vi "RT Driver VI.vi"(7 "Operation":T1, 11 "Device Reference in":T2 format="%.0x") -> (0 "Error Code":i32)   [LabVIEW 2020, in "FlexRay Custom Device Engine.lvlib"]
uses:
  FlexRay Custom Device Engine.lvlib
  <vilib>/NI VeriStand/Custom Device API/Custom Device Item Ref.ctl
  <vilib>/NI VeriStand/Custom Device API/Hardware Interface Driver VI Operation.ctl
  <vilib>/NI VeriStand/Custom Device API/Data Reference.ctl
  Shared/FREventInfo.ctl
  Shared/InterfaceState.ctl
  <vilib>/xnet/xnet.llb/XNET Control Scope.ctl
  <vilib>/NI VeriStand/Custom Device API/Global Data Refs.vi
  <vilib>/xnet/xnet.llb/XNET Read (State FlexRay Comm).vi
  <vilib>/NI VeriStand/Custom Device API/Custom Device API.lvlib
  Shared/FlexRay Custom Device Shared.lvlib
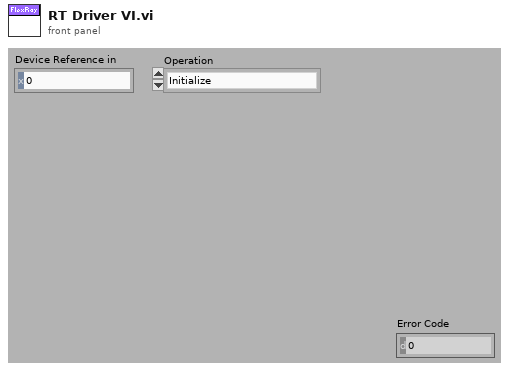
[diagram p1: front panel]
types:
  T1 = typedef "Custom Device API.lvlib/Hardware Interface Driver VI Operation.ctl" = enum16{"Initialize", "Start", "Read Data from HW", "Write Data to HW", "Close"}
  T2 = typedef "Custom Device API.lvlib/Custom Device Item Ref.ctl" = u64
  T3 = typedef "Custom Device API.lvlib/Data Reference.ctl" = i32
  T4 = typedef "FlexRay Custom Device Shared.lvlib/FREventInfo.ctl" = cluster{"Signals":refnum<k21>[], "Channel Data Ref":T3[], "Channel Data Value":dbl[]}
  T5 = typedef "FlexRay Custom Device Engine.lvlib/InterfaceState.ctl" = enum16{"Disabled", "Enabled", "Init"}
  T6 = cluster{"ctrl_stat":cluster{"ctrl_state":T2[], "FR Intf":refnum<k21>}, "FRConfig":cluster{"Write signal list":refnum<k21>[], "Output Values":dbl[], "Output Refs":T3[], "Read signal list":refnum<k21>[], "Input Values":dbl[], "Input Refs":T3[], "EventFrames list":T4[], "FR Cyclic Session":refnum<k21>, "FR Single Read Session":refnum<k21>, "FR Event Write Sessions":refnum<k21>[], "Run state":T5}, "ActiveCom":cluster{"CyclicFRActive?":bool, "EventFRActive?":bool, "IncomingFRActive?":bool}, "Device Error":errorcluster}
  T7 = typedef "XNET Control Scope.ctl" = u32
  T8 = typedef "XNET FlexRay Comm.ctl" = cluster{"fault code":i32, "fault?":bool, "FlexRay POC state":T9, "clock correction failed":u8, "passive to active count":u8, "channel A sleep?":bool, "channel B sleep?":bool}
  T9 = typedef "XNET FlexRay POC State.ctl" = u8
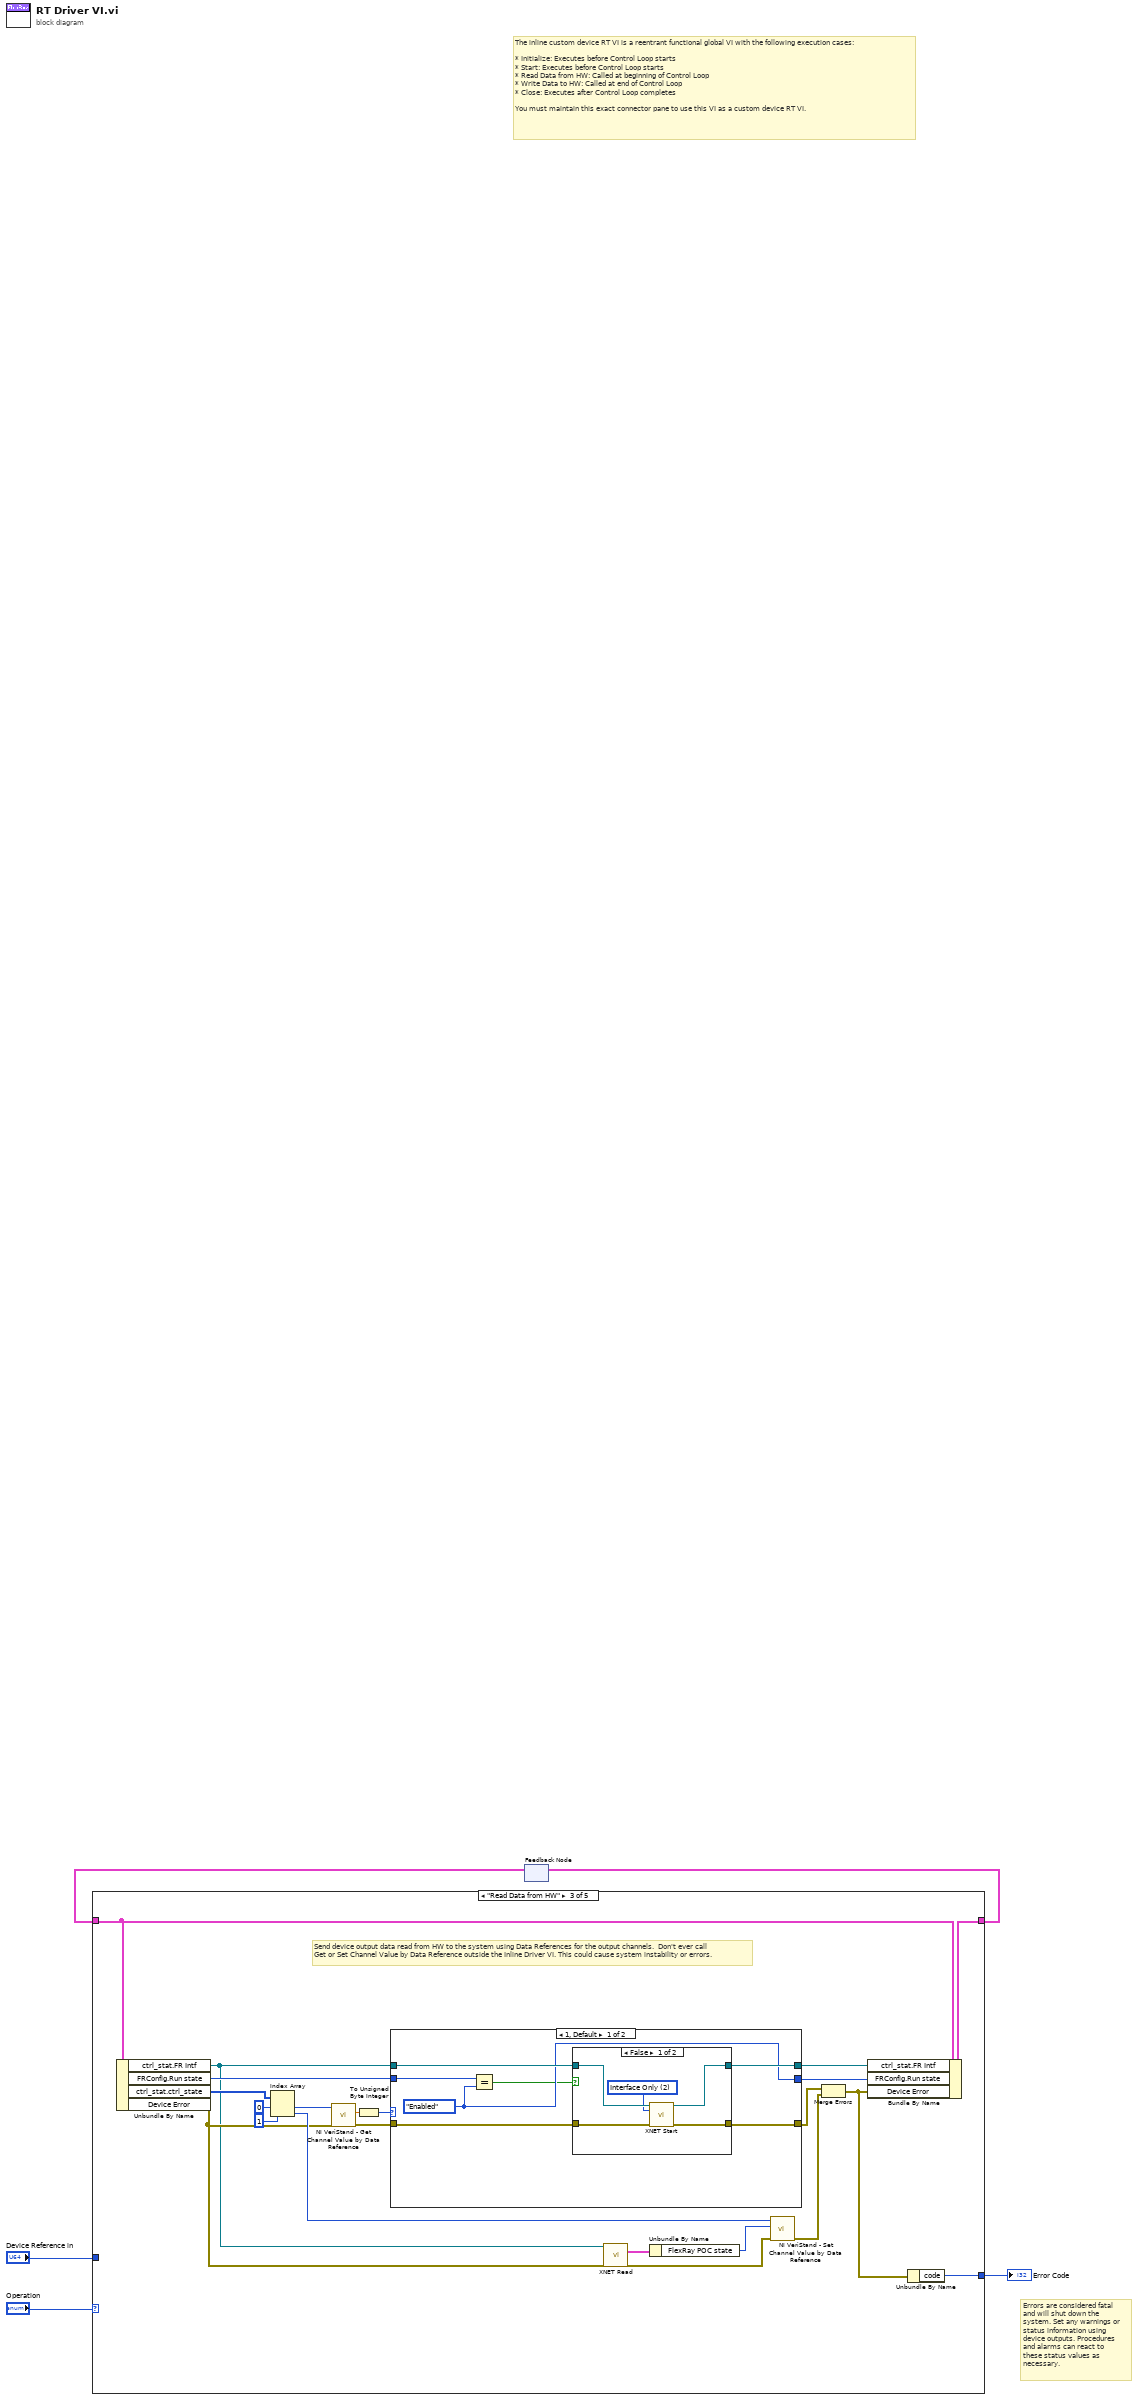
[diagram p0: block diagram]
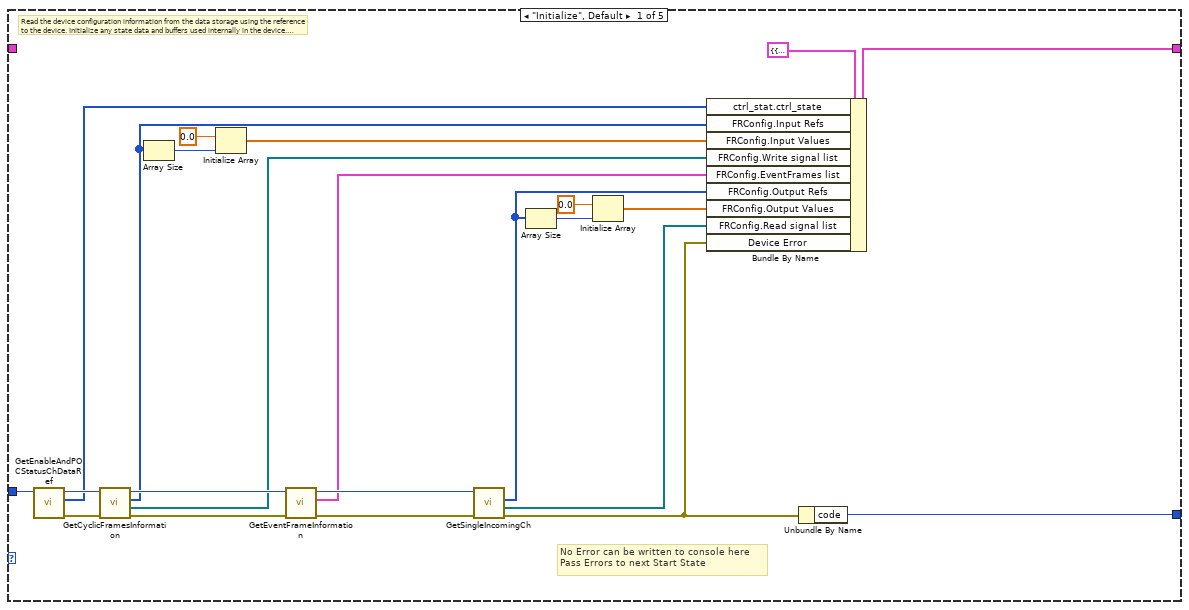
[diagram p2: hidden frame]
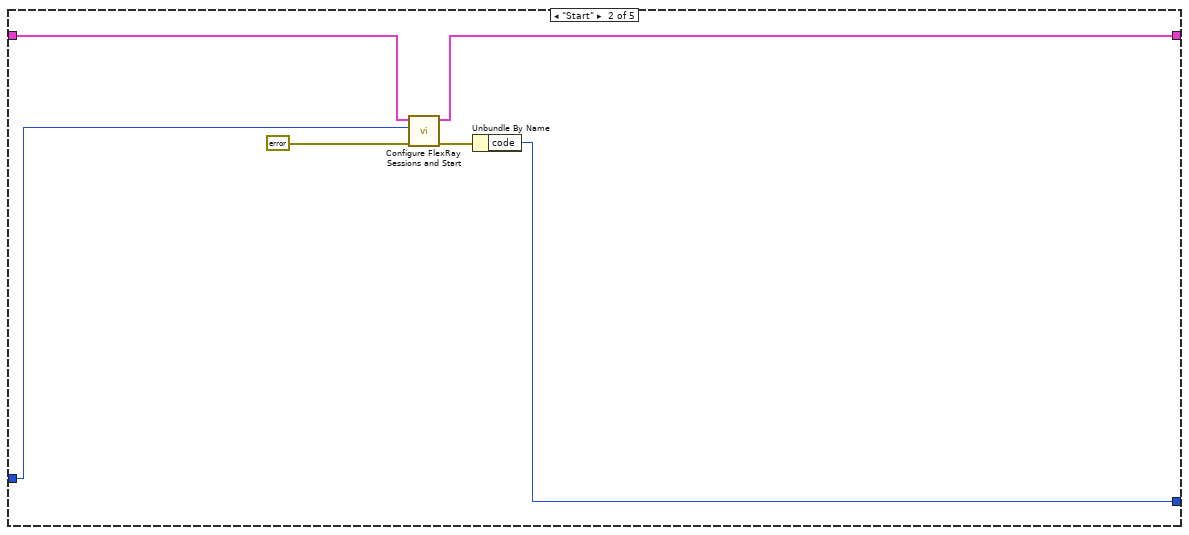
[diagram p3: hidden frame]
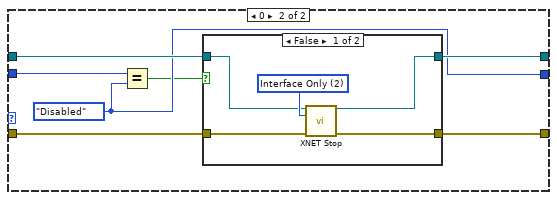
[diagram p5: hidden frame]
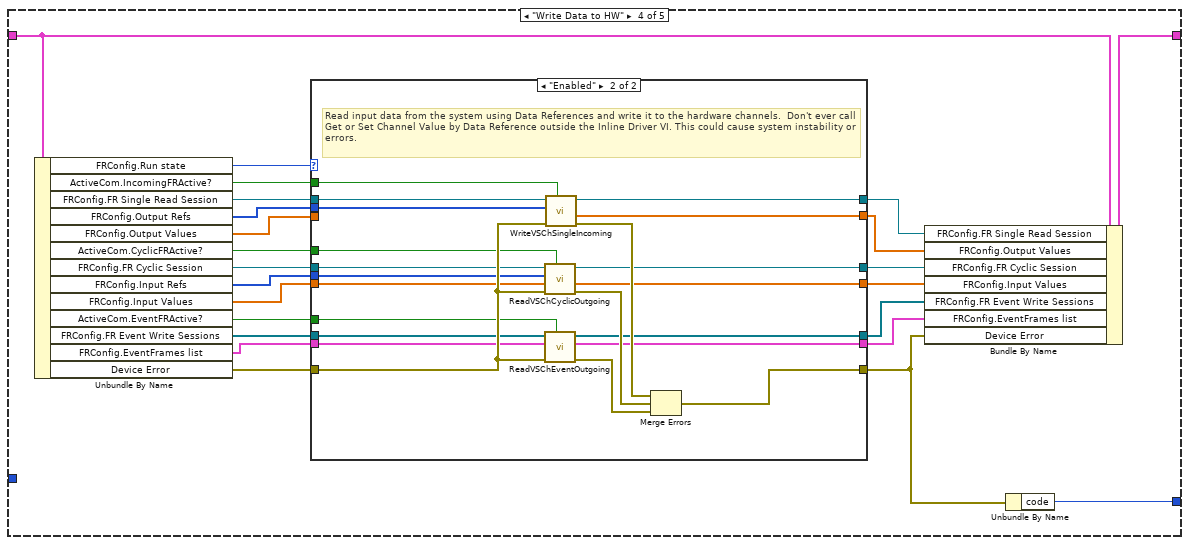
[diagram p7: hidden frame]
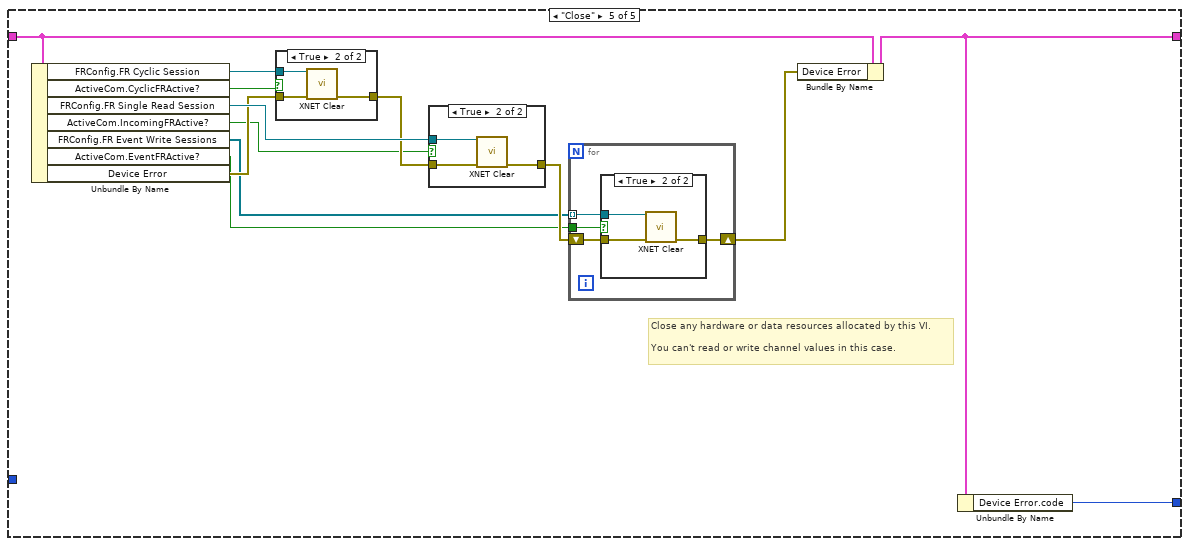
[diagram p9: hidden frame]
diagram:
  # "Errors are considered fatal and will shut down the system. Set any warnings or status information using device outputs. Procedures and alarms can react to these status values as necessary."
  # "The inline custom device RT VI is a reentrant functional global VI with the following execution cases:\n\n* Initialize: Executes before Control Loop starts\n* Start: Executes before Control Loop starts\n* Read Data from HW: Called at beginning of Control Loop\n* Write Data to HW: Called at end of Control Loop\n* Close: Executes after Control Loop completes\n\nYou must maintain this exact connector pane to use this VI as a custom device RT VI."
  n1 = feedback #1() -> (w3:T6)  [unwired: 1 out]
  n2 = case shown="\"Read Data from HW\"" "Operation" {
    tunnel: [w27 w34 w55 w106 w142] -> w4
    tunnel: w3 -> [_ w33 w56 w107 w143]
    tunnel: "Device Reference in" -> [w21 w32 _ _ _]
    tunnel: [w24 w29 w54 w104 w148] -> w1
    frame "Initialize", Default {
      # "No Error can be written to console here\nPass Errors to next Start State"
      # "Read the device configuration information from the data storage using the reference to the device. Initialize any state data and buffers used internally in the device.\n\nCompile the list of Data References for the custom device Inputs and Outputs in advance using Get Channel List and Get Channel Data Reference. Allocate any necessary data buffers and configure any state data.\n\nYou can't read or write channel values in this case."
      n3 = call "GetEnableAndPOCStatusChDataRef.vi"("Device Reference in"=w21) -> ("error out"=w20:errorcluster, "Channel Data Refs"=w16:T3[], "Device Ref out"=w17:T2)  [unwired: 8 in]
      n4 = call "GetCyclicFramesInformation.vi"("error in (no error)"=w20, "Device Ref in"=w17) -> ("error out"=w14:errorcluster, "FR Signals"=w9:refnum<k21>[], "Channel Data Ref"=w11:T3[], "Device Ref out"=w12:T2)  [unwired: 6 in]
      n5 = Array Size(array=w11) -> (size(s)=w23:i32)
      n6 = Initialize Array(0.0 ("element"), w23) -> (w10:dbl[])
      n7 = call "GetEventFrameInformation.vi"("error in (no error)"=w14, "Device Ref in"=w12) -> ("error out"=w13:errorcluster, "EventFrames"=w6:T4[], "Device Ref out"=w15:T2)  [unwired: 7 in]
      n8 = call "GetSingleIncomingCh.vi"("Device Ref in"=w15, "error in (no error)"=w13) -> ("Channel Data Ref"=w7:T3[], "FR Signals"=w18:refnum<k21>[], "error out"=w19:errorcluster)  [unwired: 5 in, 1 out]
      n9 = Array Size(array=w7) -> (size(s)=w22:i32)
      n10 = Initialize Array(0.0 ("element"), w22) -> (w8:dbl[])
      n11 = Bundle By Name(cluster=T6 {"ctrl_stat"={"ctrl_state"=[], "FR Intf"=""}, "FRConfig"={"Write signal list"=[], "Output Values"=[], "Output Refs"=[], "Read signal list"=[], "Input Values"=[], "Input Refs"=[], "EventFrames list"=[], "FR Cyclic Session"="", "FR Single Read Session"="", "FR Event Write Sessions"=[], "Run state"=enum."Init"}, "ActiveCom"={"CyclicFRActive?"=FALSE, "EventFRActive?"=FALSE, "IncomingFRActive?"=FALSE}, "Device Error"={"status"=FALSE, "code"=0, "source"=""}}, "ctrl_stat.ctrl_state"=w16, "FRConfig.Input Refs"=w11, "FRConfig.Input Values"=w10, "FRConfig.Write signal list"=w9, "FRConfig.EventFrames list"=w6, "FRConfig.Output Refs"=w7, "FRConfig.Output Values"=w8, "FRConfig.Read signal list"=w18, "Device Error"=w19) -> (w27:T6)
      n12 = Unbundle By Name(w19) -> ("code"=w24:i32)
    }
    frame "Start" {
      n13 = call "Configure FlexRay Sessions and Start.vi"("error in (no error)"=errorcluster {"status"=FALSE, "code"=0, "source"=""}, "Device Reference in"=w32, "cluster in"=w33) -> ("error out"=w30:errorcluster, "cluster out"=w34:T6)  [unwired: 7 in]
      n14 = Unbundle By Name(w30) -> ("code"=w29:i32)
    }
    frame "Read Data from HW" {
      # "Send device output data read from HW to the system using Data References for the output channels.  Don't ever call Get or Set Channel Value by Data Reference outside the Inline Driver VI. This could cause system instability or errors."
      n15 = Unbundle By Name(w56) -> ("ctrl_stat.FR Intf"=w37:refnum<k21>, "FRConfig.Run state"=w44:T5, "ctrl_stat.ctrl_state"=w53:T2[], "Device Error"=w39:errorcluster)
      n16 = Index Array(array=w53, index #1=0, index #2=1 ("index")) -> (element #1=w51:T2, element #2=w42:T2)
      n17 = call <vilib>:"NI VeriStand - Get Channel Value by Data Reference.vi"("error in (no error)"=w39, "Data Reference in"=w51) -> ("error out"=w48:errorcluster, "Value"=w50:dbl)  [unwired: 8 in]
      n18 = To Unsigned Byte Integer(number=w50) -> (unsigned 8bit integer=w49:u8)
      n19 = case shown="1, Default" w49 {
        tunnel: w48 -> [w63 w77]
        tunnel: [w60 w76] -> w47
        tunnel: [w62 w75] -> w46
        tunnel: w37 -> [w61 w74]
        tunnel: [w58 w72] -> w45
        tunnel: w44 -> [w59 w73]
        frame 1, Default {
          w58 = InterfaceState."Enabled" ("FRConfig.Run state")
          n20 = Equal?(x=w59, y=w58) -> (x = y?=w57:bool)
          n21 = case shown="False" w57 {
            tunnel: w63 -> [w68 w69]
            tunnel: [w67 w69] -> w62
            tunnel: w61 -> [w66 w70]
            tunnel: [w64 w70] -> w60
            frame False {
              w65 = T7 2 items=["Normal", "Session Only", "Interface Only", "Session Only Blocking"] ("scope (normal)")
              n22 = call <vilib>:"XNET Start.vi"("session in"=w66, "scope (normal)"=w65, "error in (no error)"=w68) -> ("session out"=w64:refnum<k21>, "error out"=w67:errorcluster)  [unwired: 11 in]
            }
            frame True {
            }
          }
        }
        frame 0 {
          w72 = InterfaceState."Disabled" ("FRConfig.Run state")
          n23 = Equal?(x=w73, y=w72) -> (x = y?=w71:bool)
          n24 = case shown="False" w71 {
            tunnel: w77 -> [w82 w83]
            tunnel: [w80 w84] -> w76
            tunnel: [w79 w83] -> w75
            tunnel: w74 -> [w78 w84]
            frame False {
              w81 = T7 2 items=["Normal", "Session Only", "Interface Only", "Session Only Blocking"] ("scope (normal)")
              n25 = call <vilib>:"XNET Stop.vi"("session in"=w78, "scope (normal)"=w81, "error in (no error)"=w82) -> ("session out"=w80:refnum<k21>, "error out"=w79:errorcluster)  [unwired: 11 in]
            }
            frame True {
            }
          }
        }
      }
      n26 = call-poly <vilib>:"XNET Read.vi"("session in"=w37, "error in (no error)"=w39) -> ("FlexRay comm"=w40:T8, "error out"=w38:errorcluster)  [unwired: 11 in, 1 out]
      n27 = Unbundle By Name(w40) -> ("FlexRay POC state"=w36:T9)
      n28 = call <vilib>:"NI VeriStand - Set Channel Value by Data Reference.vi"("error in (no error)"=w38, "Value"=w36, "Data Reference in"=w42) -> ("error out"=w35:errorcluster)  [unwired: 8 in]
      n29 = Merge Errors(w46, w35) -> (w41:errorcluster)
      n30 = Bundle By Name(cluster=w56, "ctrl_stat.FR Intf"=w47, "FRConfig.Run state"=w45, "Device Error"=w41) -> (w55:T6)
      n31 = Unbundle By Name(w41) -> ("code"=w54:i32)
    }
    frame "Write Data to HW" {
      n32 = Unbundle By Name(w107) -> ("FRConfig.Run state"=w97:T5, "ActiveCom.IncomingFRActive?"=w88:bool, "FRConfig.FR Single Read Session"=w89:refnum<k21>, "FRConfig.Output Refs"=w98:T3[], "FRConfig.Output Values"=w103:dbl[], "ActiveCom.CyclicFRActive?"=w100:bool, "FRConfig.FR Cyclic Session"=w91:refnum<k21>, "FRConfig.Input Refs"=w96:T3[], "FRConfig.Input Values"=w105:dbl[], "ActiveCom.EventFRActive?"=w95:bool, "FRConfig.FR Event Write Sessions"=w90:refnum<k21>[], "FRConfig.EventFrames list"=w94:T4[], "Device Error"=w102:errorcluster)
      n33 = case shown="\"Enabled\"" w97 {
        tunnel: w105 -> [w111 w124]
        tunnel: [w111 w127] -> w86
        tunnel: w103 -> [w109 _]
        tunnel: [w109 w126] -> w87
        tunnel: w102 -> [w113 w129]
        tunnel: [w113 w134] -> w101
        tunnel: w96 -> [_ w123]
        tunnel: w89 -> [w114 w132]
        tunnel: w100 -> [_ w121]
        tunnel: [w114 w131] -> w99
        tunnel: [w110 w130] -> w93
        tunnel: w98 -> [_ w122]
        tunnel: [w112 w117] -> w92
        tunnel: w95 -> [_ w119]
        tunnel: w94 -> [w108 w116]
        tunnel: w91 -> [w110 w120]
        tunnel: w88 -> [_ w125]
        tunnel: w90 -> [w112 w118]
        tunnel: [w108 w115] -> w85
        frame "Disabled", Default {
          # "Should it be 0"
        }
        frame "Enabled" {
          # "Read input data from the system using Data References and write it to the hardware channels.  Don't ever call Get or Set Channel Value by Data Reference outside the Inline Driver VI. This could cause system instability or errors."
          n34 = call "ReadVSChCyclicOutgoing.vi"("CyclicFRActive?"=w121, "error in (no error)"=w129, "Input Values in"=w124, "Input Refs"=w123, "Refnum in"=w120) -> ("error out"=w133:errorcluster, "Input Values out"=w127:dbl[], "Refnum out"=w130:refnum<k21>)  [unwired: 4 in]
          n35 = call "ReadVSChEventOutgoing.vi"("EventFRActive?"=w119, "error in (no error)"=w129, "EventFrames list"=w116, "Refnum in"=w118) -> ("error out"=w128:errorcluster, "EventFrames list Out"=w115:T4[], "Refnum out"=w117:refnum<k21>[])  [unwired: 5 in]
          n36 = call "WriteVSChSingleIncoming.vi"("IncomingFRActive?"=w125, "error in (no error)"=w129, "Output Refs"=w122, "Refnum in"=w132) -> ("error out"=w135:errorcluster, "data"=w126:dbl[], "Refnum out"=w131:refnum<k21>)  [unwired: 5 in]
          n37 = Merge Errors(w135, w133, w128) -> (w134:errorcluster)
        }
      }
      n38 = Bundle By Name(cluster=w107, "FRConfig.FR Single Read Session"=w99, "FRConfig.Output Values"=w87, "FRConfig.FR Cyclic Session"=w93, "FRConfig.Input Values"=w86, "FRConfig.FR Event Write Sessions"=w92, "FRConfig.EventFrames list"=w85, "Device Error"=w101) -> (w106:T6)
      n39 = Unbundle By Name(w101) -> ("code"=w104:i32)
    }
    frame "Close" {
      # "Close any hardware or data resources allocated by this VI.\n\nYou can't read or write channel values in this case."
      n40 = Unbundle By Name(w143) -> ("FRConfig.FR Cyclic Session"=w147:refnum<k21>, "ActiveCom.CyclicFRActive?"=w138:bool, "FRConfig.FR Single Read Session"=w146:refnum<k21>, "ActiveCom.IncomingFRActive?"=w137:bool, "FRConfig.FR Event Write Sessions"=w140:refnum<k21>[], "ActiveCom.EventFRActive?"=w136:bool, "Device Error"=w144:errorcluster)
      n41 = case shown="True" w138 {
        tunnel: w147 -> [_ w164]
        tunnel: [w161 w163] -> w145
        tunnel: w144 -> [w161 w162]
        frame False {
        }
        frame True {
          n42 = call <vilib>:"XNET Clear.vi"("session in"=w164, "error in (no error)"=w162) -> ("error out"=w163:errorcluster)  [unwired: 13 in]
        }
      }
      n43 = case shown="True" w137 {
        tunnel: w146 -> [_ w160]
        tunnel: w145 -> [w157 w159]
        tunnel: [w157 w158] -> w141
        frame False {
        }
        frame True {
          n44 = call <vilib>:"XNET Clear.vi"("session in"=w160, "error in (no error)"=w159) -> ("error out"=w158:errorcluster)  [unwired: 13 in]
        }
      }
      n45 = for {
        tunnel: w140 -> [w151] mode=indexing
        tunnel: w136 -> [w149]
        shift-right: [w150] -> w139
        shift-left: w141 -> [w152]
        n46 = case shown="True" w149 {
          tunnel: w152 -> [w153 w156]
          tunnel: w151 -> [_ w154]
          tunnel: [w153 w155] -> w150
          frame False {
          }
          frame True {
            n47 = call <vilib>:"XNET Clear.vi"("session in"=w154, "error in (no error)"=w156) -> ("error out"=w155:errorcluster)  [unwired: 13 in]
          }
        }
      }
      n48 = Bundle By Name(cluster=w143, "Device Error"=w139) -> (w142:T6)
      n49 = Unbundle By Name(w142) -> ("Device Error.code"=w148:i32)
    }
  }
  "Error Code" <- w1
  n50 = feedback-in #1(w4) -> ()
